vi "NIVEL DE TANQUE.vi"() -> ()   [LabVIEW 2019]
panel:
  in  "Accion":bool
  in  "Vaciado/LLenado":bool
  in  "Velocidad":bool
  out "Tanque Vacio":bool
  out "Tanque LLeno":bool
  out "Paro":bool
  out "Vaciando":bool
  out "Llenando":bool
  out "Tanque":dbl(slide) scale=0.0..1000.0
  # "ALTA"
  # "BAJA"
  # "CONTINUAR"
  # "LLENAR"
  # "PARAR"
  # "VACIAR"
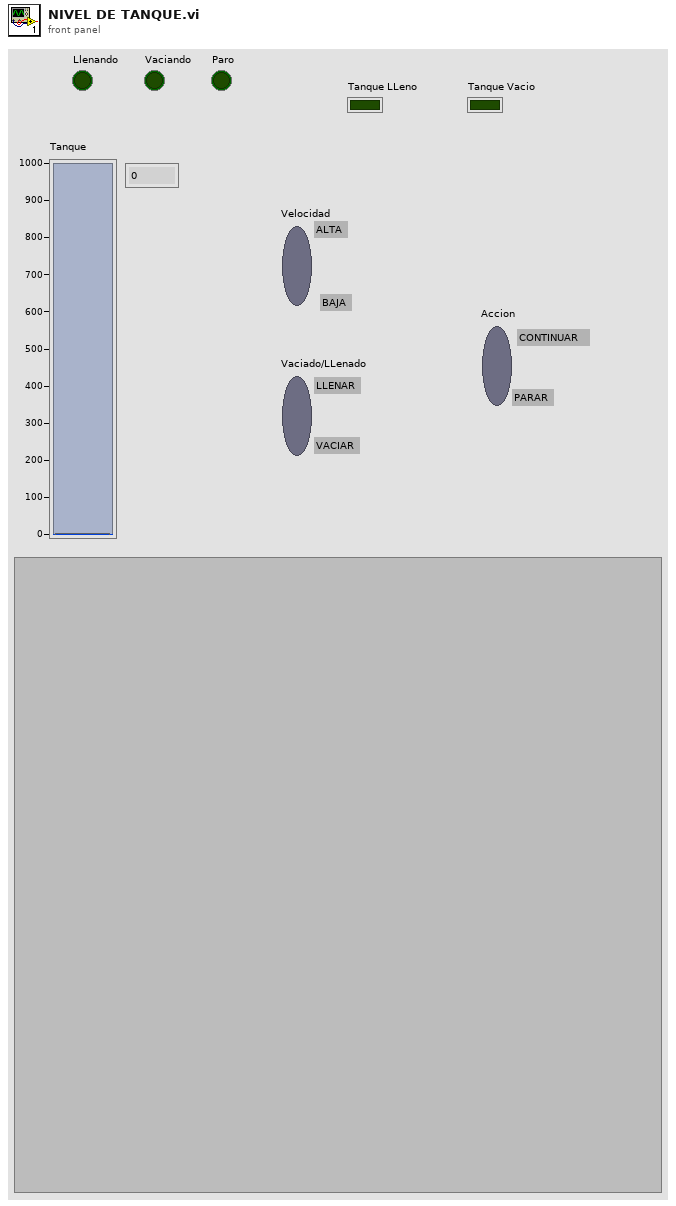
[diagram p1: front panel]
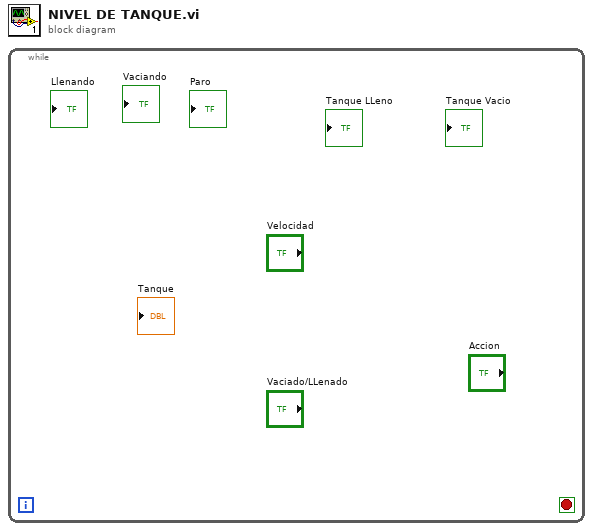
[diagram p0: block diagram]
diagram:
  n1 = while {
    stop <- _ stop-if-true
  }
